vi "Service layer time.vi"(8 "error in (no error)":errorcluster, 9 "time config":T1, 10 "ADiagModuleIndex":i32, 11 "路径输入":path) -> (0 "error out":errorcluster, 2 "returns":i32[](array[numeric]), 3 "路径输出":path)   [LabVIEW 2014]
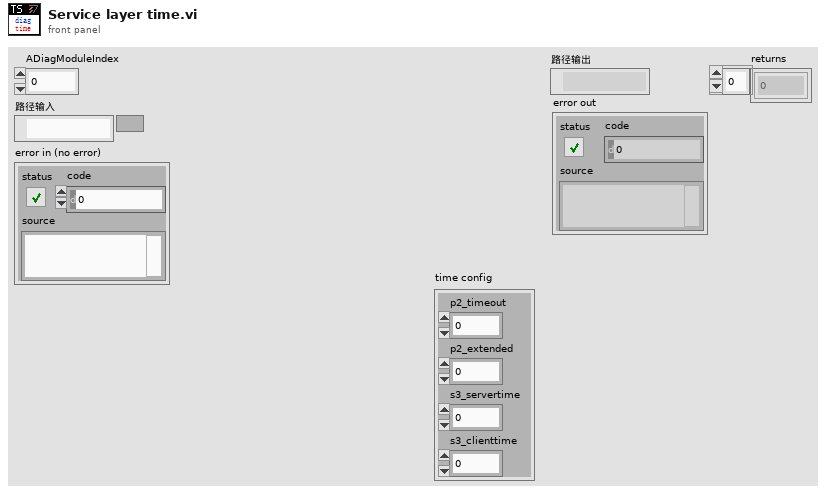
[diagram p1: front panel]
types:
  T1 = cluster{"p2_timeout":i32, "p2_extended":i32, "s3_servertime":i32, "s3_clienttime":i32}
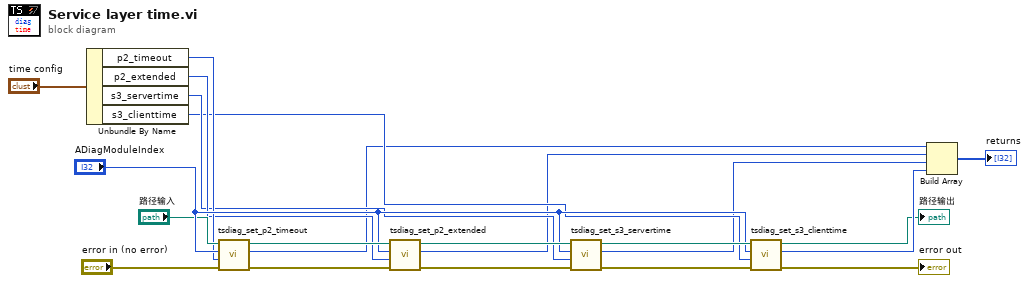
[diagram p0: block diagram]
diagram:
  n1 = Unbundle By Name("time config") -> ("p2_timeout"=w11:i32, "p2_extended"=w10:i32, "s3_servertime"=w9:i32, "s3_clienttime"=w8:i32)
  n2 = call "tsdiag_set_p2_timeout.vi"("error in (no error)"="error in (no error)", "ATimeMs"=w11, "ADiagModuleIndex"="ADiagModuleIndex", "路径输入"="路径输入") -> ("error out"=w20:errorcluster, "return"=w7:i32, "路径输出"=w21:path)  [unwired: 5 in]
  n3 = call "tsdiag_set_p2_extended.vi"("error in (no error)"=w20, "ATimeMs"=w10, "ADiagModuleIndex"="ADiagModuleIndex", "路径输入"=w21) -> ("error out"=w18:errorcluster, "return"=w6:i32, "路径输出"=w19:path)  [unwired: 5 in]
  n4 = call "tsdiag_set_s3_servertime.vi"("error in (no error)"=w18, "ATimeMs"=w9, "ADiagModuleIndex"="ADiagModuleIndex", "路径输入"=w19) -> ("error out"=w16:errorcluster, "return"=w5:i32, "路径输出"=w17:path)  [unwired: 5 in]
  n5 = call "tsdiag_set_s3_clienttime.vi"("error in (no error)"=w16, "ATimeMs"=w8, "ADiagModuleIndex"="ADiagModuleIndex", "路径输入"=w17) -> ("error out"=→"error out":errorcluster, "return"=w4:i32, "路径输出"=→"路径输出":path)  [unwired: 5 in]
  n6 = Build Array(w7, w6, w5, w4) -> (→"returns":i32[])
